vi "Set_Tunnel_Speed.vi"(3 "Mode":T1, 5 "Tunnel Velocity m/s":dbl min=0.0 max=50.0 format="%.2f") -> (0 "Error String":string, 2 "Max allowable Tunnel Velocity":dbl)   [LabVIEW 2017]
doc: "This is an example of using features of the VI Server as a client. It shows how you might browse from one or more applications that may be exporting data from one or more data stations. \n\nThe example shows how to query a server for its list of exported VIs, how to get references to the VIs, and how call them with the Call By Reference function."
uses:
  Sub VIs/ADAM Controls/Tunnel_speed_mode.ctl
  Anemometry/Anemometry Sub Vis/File/Setup_Filetype.ctl
  Sub VIs/ADAM Controls/Update_scan_value.ctl
  Anemometry/Anemometry Sub Vis/Controls/Global_mode.ctl
  Sub VIs/ADAM Controls/Ch_description_ADAM.ctl
  Sub VIs/ADAM Controls/Module_type_ADAM.ctl
  Sub VIs/ADAM Controls/Function_ADAM.ctl
  Sub VIs/ADAM Controls/Channel_State.ctl
  Sub VIs/ADAM Controls/Calib_type_ADAM.ctl
  Sub VIs/ADAM Controls/Address.ctl
  <vilib>/Analysis/baseanly.llb/Mean (DBL).vi
  Anemometry/Anemometry Sub Vis/Globals/Preference_global.vi
  Anemometry/Anemometry Sub Vis/Globals/Trav_pos_global.vi
  Anemometry/Anemometry Sub Vis/Globals/Constants_global.vi
  <vilib>/Analysis/NI_AALBase.lvlib
panel:
  in  "Set EnFlo Tun Speed":refnum<vi>
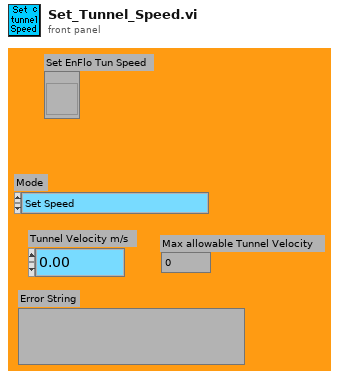
[diagram p1: front panel]
types:
  T1 = typedef "Tunnel_speed_mode.ctl" = enum16{"Set Speed", "Set Speed then wait", "Is tunnel speed allowable?"}
  T2 = typedef "Setup_Filetype.ctl" = enum16{"Measurement Setups", "Calibration Setups", "General", "Results File Plotter Setups", "Speed Calib Tweaks"}
  T3 = typedef "Channel_State.ctl" = enum16{"On", "Off", "Always On", "Always Off"}
  T4 = typedef "Calib_type_ADAM.ctl" = string
  T5 = typedef "Module_type_ADAM.ctl" = string
  T6 = typedef "Ch_description_ADAM.ctl" = cluster{"Ch Name":string, "Type":T5, "Function":T7, "Ch State":T3, "Calibration type":T4, "A":dbl, "B":dbl, "C":dbl, "D":dbl, "Comments":string, "Address":T8, "String":string, "Duty":u16}
  T7 = typedef "Function_ADAM.ctl" = enum16{"Analogue Input", "Digital Input", "Event counter", "Event rate", "Analogue Output", "Digital Output", "Relay Output"}
  T8 = typedef "Address.ctl" = cluster{"Main":i32, "Ch.":i32, "Sub":i32, "Port Name":string}
  T9 = typedef "Global_mode.ctl" = enum16{"Read Global", "Load Global From File", "Write Global to File"}
  T10 = typedef "Update_scan_value.ctl" = cluster{"Channel Name":string, "New Value":dbl}
  T11 = typedef "Server_Comms.ctl" = enum16{"Server Link Healthy", "Do Not Link To Server"}
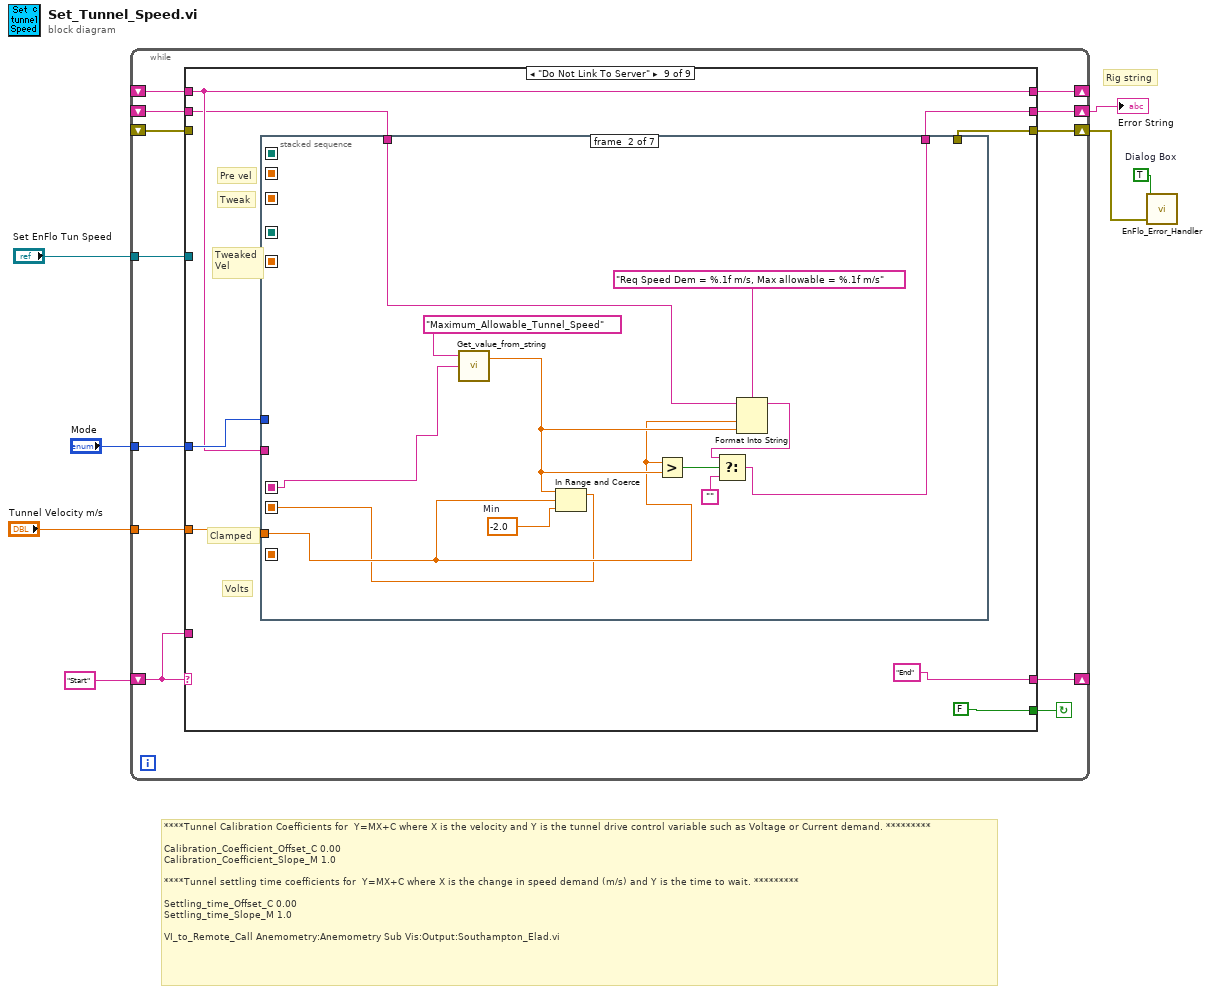
[diagram p0: block diagram]
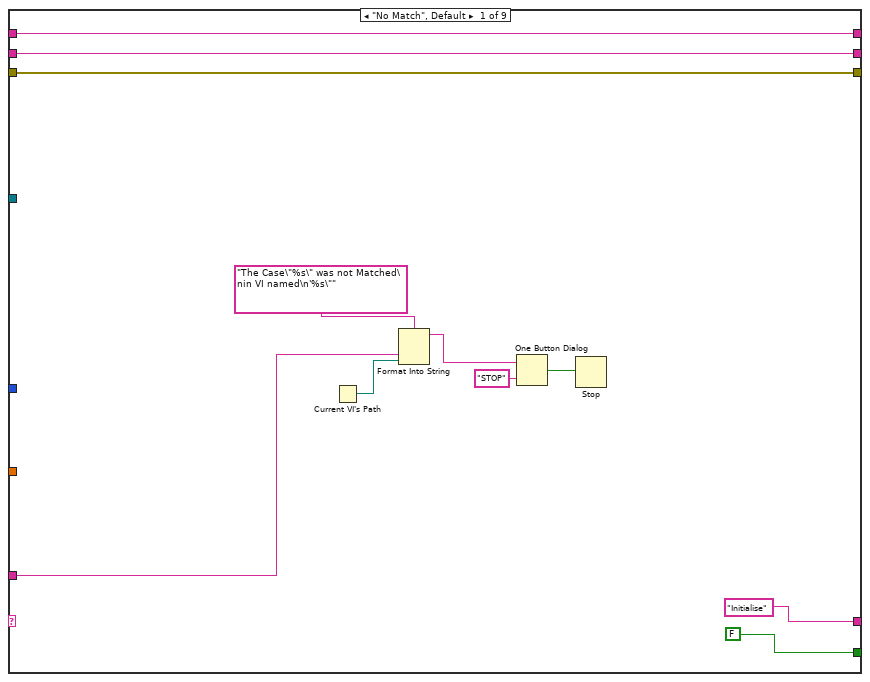
[diagram p2: hidden frame]
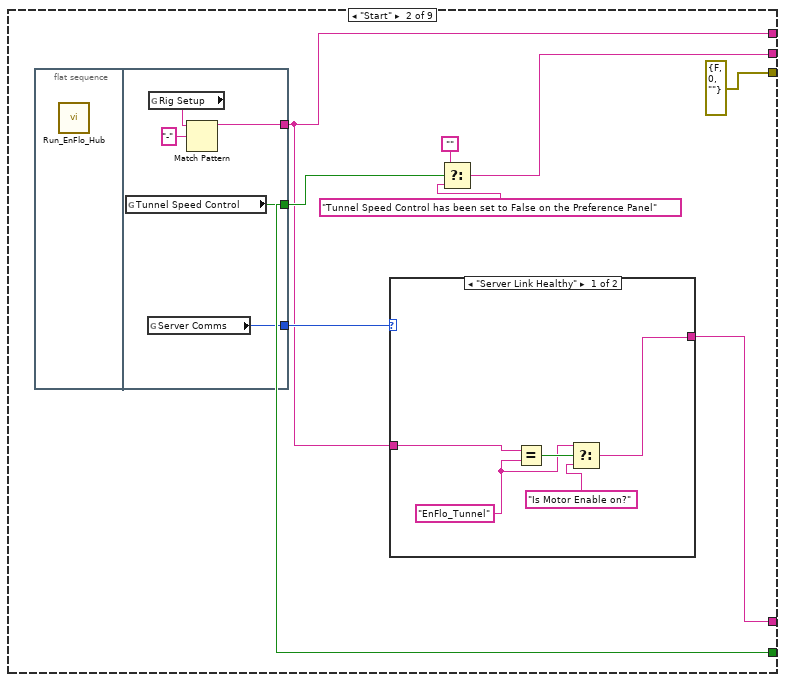
[diagram p3: hidden frame]
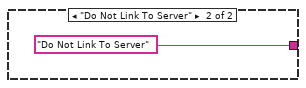
[diagram p4: hidden frame]
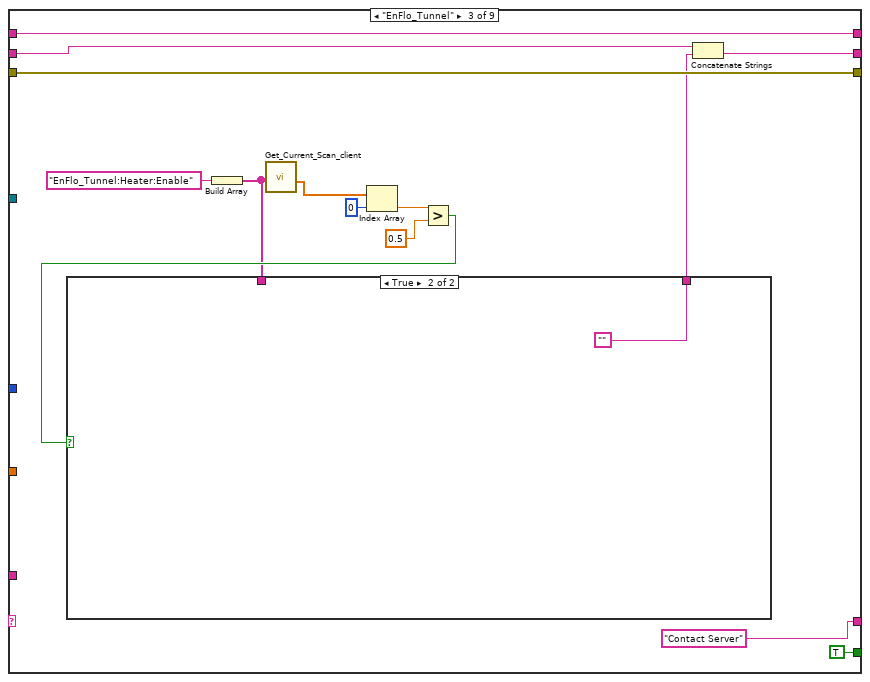
[diagram p5: hidden frame]
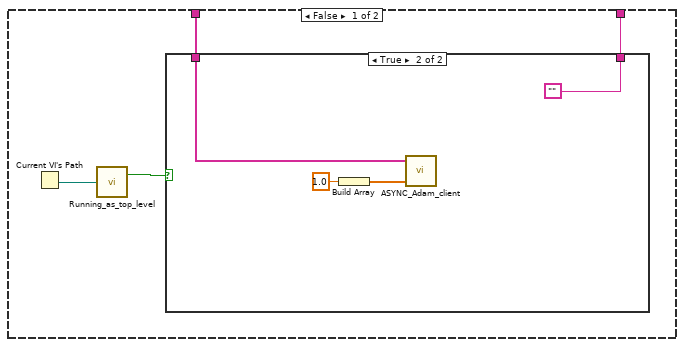
[diagram p6: hidden frame]
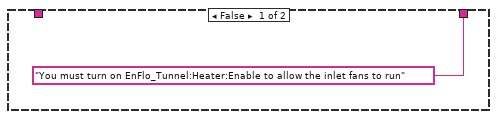
[diagram p7: hidden frame]
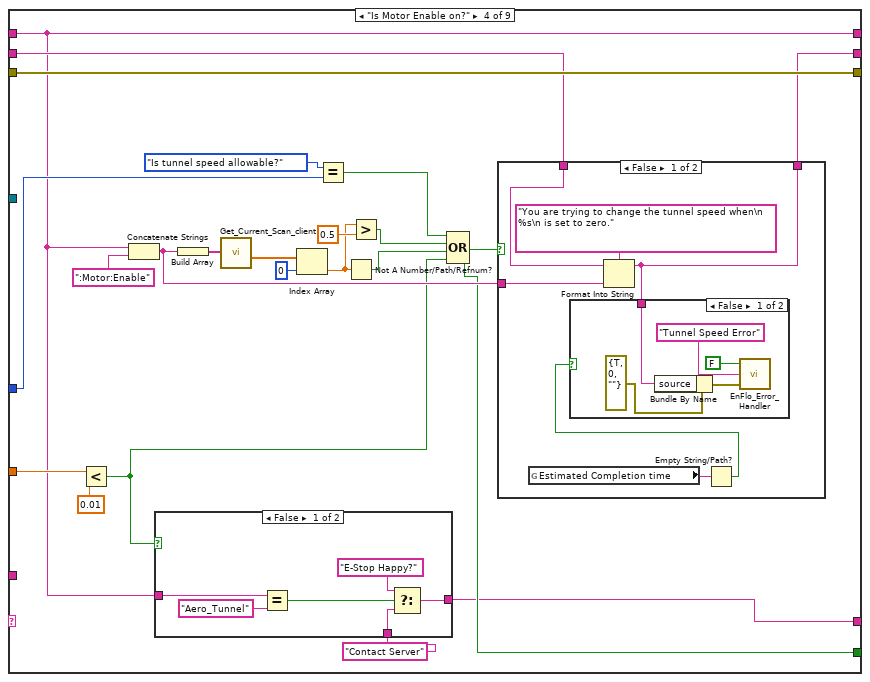
[diagram p8: hidden frame]
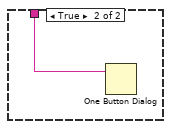
[diagram p10: hidden frame]
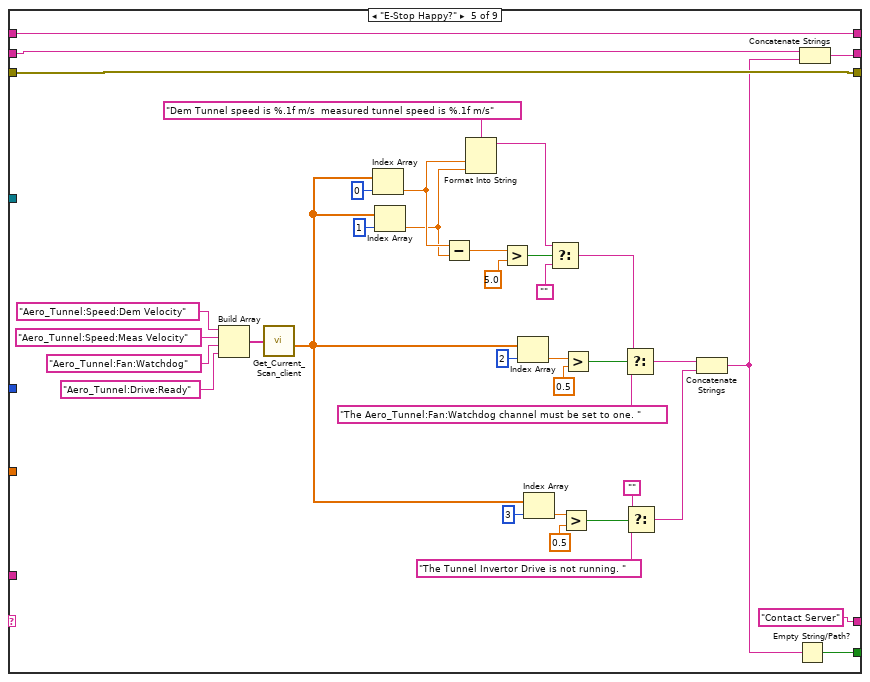
[diagram p12: hidden frame]
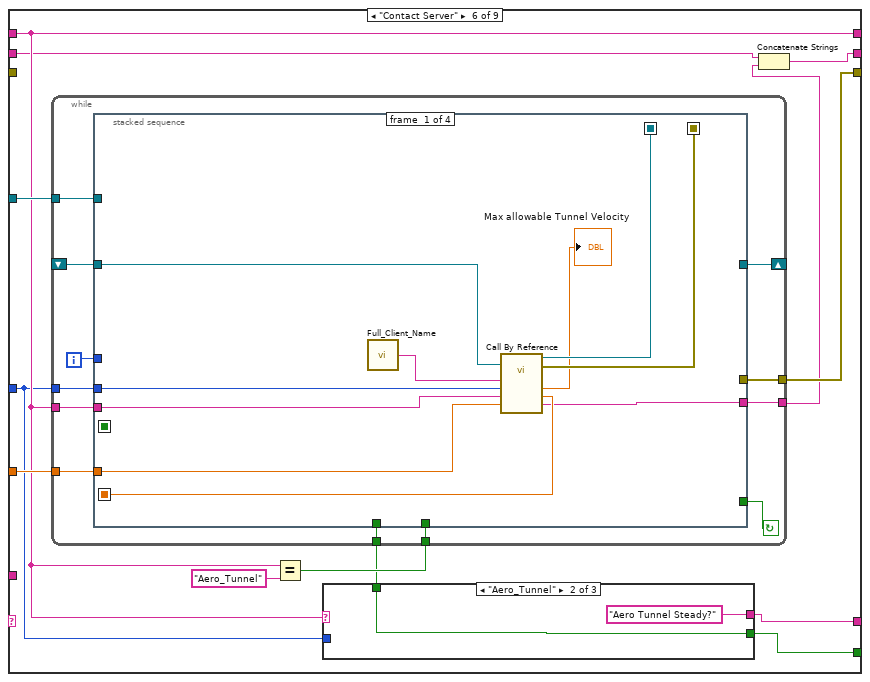
[diagram p13: hidden frame]
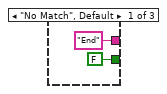
[diagram p14: hidden frame]
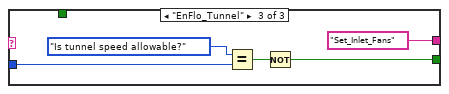
[diagram p15: hidden frame]
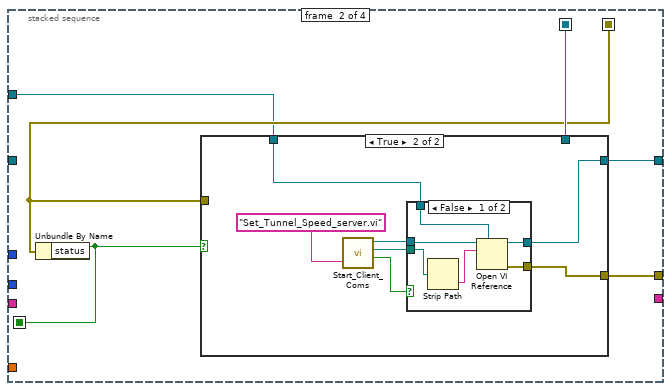
[diagram p16: hidden frame]
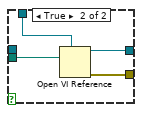
[diagram p18: hidden frame]
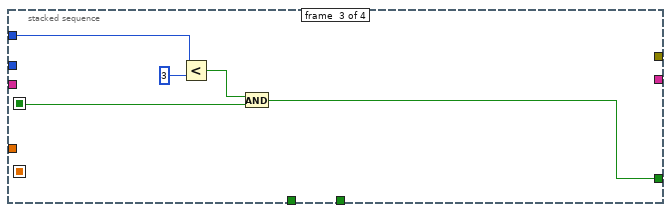
[diagram p19: hidden frame]
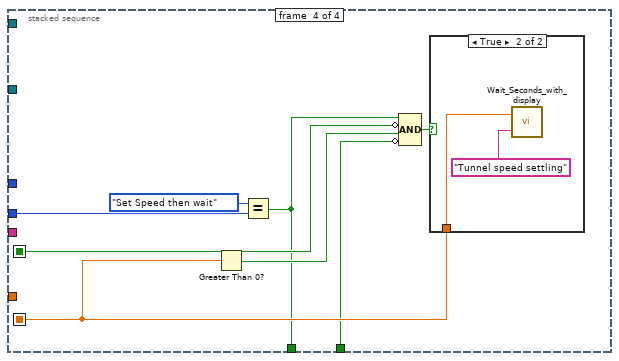
[diagram p20: hidden frame]
diagram:
  w7 = TRUE  # Dialog Box
  # "Rig string"
  # "****Tunnel Calibration Coefficients for  Y=MX+C where X is the velocity and Y is the tunnel drive control variable such as Voltage or Current demand. *********\n\nCalibration_Coefficient_Offset_C\t0.00\nCalibration_Coefficient_Slope_M\t1.0\n\n****Tunnel settling time coefficients for  Y=MX+C where X is the change in speed demand (m/s) and Y is the time to wait. *********\n\nSettling_time_Offset_C\t0.00\nSettling_time_Slope_M\t1.0\n\nVI_to_Remote_Call\tAnemometry:Anemometry Sub Vis:Output:Southampton_Elad.vi"
  n1 = while {
    shift-left: "Start" -> [w18]
    shift-right: [w19] -> _
    shift-right: [w17] -> w5
    shift-left: _ -> [w16]
    shift-right: [w15] -> w4
    shift-left: _ -> [w10]
    tunnel: "Mode" -> [w14]
    tunnel: "Tunnel Velocity m/s" -> [w13]
    shift-right: [w12] -> _
    shift-left: _ -> [w11]
    tunnel: "Set EnFlo Tun Speed" -> [w8]
    stop <- w9 continue-if-true
    n2 = case shown="\"Do Not Link To Server\"" w18 {
      tunnel: [FALSE w36 TRUE ("Tunnel Speed Control") w81 w129 w158 w242 FALSE ("Tunnel Speed Control") FALSE] -> w9
      tunnel: ["Initialise" w32 "Contact Server" ("f") w74 "Contact Server" ("f") w157 "Aero Tunnel Steady?" ("f") "End" ("f") "End"] -> w19
      tunnel: w18 -> [w25 _ _ _ _ _ _ _ _]
      tunnel: [w22 w34 w52 w83 w143 w153 w258 w285 w300] -> w17
      tunnel: w16 -> [w22 _ w54 w82 w144 w154 w258 w285 w297]
      tunnel: [w20 errorcluster {"status"=FALSE, "code"=0, "source"=""} ("error out") w55 w85 w138 w164 w257 w284 w299] -> w15
      tunnel: w14 -> [_ _ _ w79 _ w156 _ _ w302]
      tunnel: w13 -> [_ _ _ w86 _ w165 w249 w266 w301]
      tunnel: [w21 w31 w63 w77 w152 w159 w259 w286 w298] -> w12
      tunnel: w11 -> [w21 _ w63 w77 w152 w159 w259 w286 w298]
      tunnel: w10 -> [w20 _ w55 w85 w138 _ w257 w284 _]
      tunnel: w8 -> [_ _ _ _ _ w163 _ _ _]
      frame "No Match", Default {
        n3 = Current VI's Path() -> (path=w24:path)
        n4 = Format Into String(format string="The Case\"%s\" was not Matched\nin VI named\n'%s\"" ("Format String"), w25, w24) -> (resulting string=w28:string)  [unwired: 2 in, 1 out]
        n5 = One Button Dialog(message=w28, button name ("OK")="STOP") -> (true=w26:bool)
        n6 = Stop(stop? (T)=w26) -> ()
      }
      frame "Start" {
        n7 = flat-sequence {
          tunnel: [w49] -> w38
          tunnel: [w48] -> w36
          tunnel: [w45] -> w31
          frame #0 {
            n8 = call "Run_EnFlo_Hub.vi"() -> ()  [unwired: 1 in, 7 out]
          }
          frame #1 {
            n9 = global read "Preference_global.vi" "Tunnel Speed Control"() -> (w48:bool)
            n10 = global read "Preference_global.vi" "Server Comms"() -> (w49:T11)
            n11 = global read "Preference_global.vi" "Rig Setup"() -> (w47:string)
            n12 = Match Pattern(string=w47, regular expression="-") -> (before substring=w45:string)  [unwired: 4 out]
          }
        }
        n13 = case shown="\"Server Link Healthy\"" w38 {
          tunnel: [w40 "Do Not Link To Server"] -> w32
          tunnel: w31 -> [w43 _]
          frame "Server Link Healthy" {
            w39 = "EnFlo_Tunnel"
            n14 = Equal?(x=w43, y=w39) -> (x = y?=w42:bool)
            n15 = Select(t=w39, s=w42, f="Is Motor Enable on?") -> (s? t:f=w40:string)
          }
          frame "Do Not Link To Server" {
          }
        }
        n16 = Select(t="", s=w36, f="Tunnel Speed Control has been set to False on the Preference Panel" ("Error String")) -> (s? t:f=w34:string)
      }
      frame "EnFlo_Tunnel" {
        n17 = Build Array("EnFlo_Tunnel:Heater:Enable") -> (w56:string[])
        n18 = call "Get_Current_Scan_client.vi"("ADAM Ch Names"=w56) -> ("Numerical Values"=w61:dbl[])  [unwired: 3 out]
        n19 = Index Array(array=w61, index=0) -> (element=w59:dbl)
        n20 = Greater?(x=w59, y=0.5) -> (0:w57:bool)
        n21 = case shown="True" w57 {
          tunnel: w56 -> [w65 _]
          tunnel: [w64 ""] -> w53
          frame False {
            n22 = Current VI's Path() -> (path=w67:path)
            n23 = call "Running_as_top_level.vi"("Vi path name"=w67) -> ("Top Level"=w66:bool)  [unwired: 1 out]
            n24 = case shown="True" w66 {
              tunnel: w65 -> [_ w71]
              tunnel: ["You must turn on EnFlo_Tunnel:Heater:Enable to allow the inlet fans to run" ""] -> w64
              frame False {
              }
              frame True {
                n25 = Build Array(1.0 ("element")) -> (w72:dbl[])
                n26 = call "ASYNC_Adam_client.vi"("Values"=w72, "Channel Names"=w71) -> ()  [unwired: 1 in, 2 out]
              }
            }
          }
          frame True {
          }
        }
        n27 = Concatenate Strings(w54, w53) -> (w52:string)
      }
      frame "Is Motor Enable on?" {
        n28 = Less?(x=w86, y=0.01) -> (x < y?=w76:bool)
        n29 = Concatenate Strings(w77, ":Motor:Enable" ("string")) -> (w84:string)
        n30 = case shown="False" w76 {
          tunnel: w77 -> [w100 _]
          tunnel: [w98 w102] -> w74
          tunnel: "Contact Server" ("f") -> [w96 w102]
          frame False {
            n31 = Equal?(x=w100, y="Aero_Tunnel") -> (x = y?=w99:bool)
            n32 = Select(t="E-Stop Happy?" ("f"), s=w99, f=w96) -> (s? t:f=w98:string)
          }
          frame True {
          }
        }
        n33 = Build Array(w84) -> (w88:string[])
        n34 = call "Get_Current_Scan_client.vi"("ADAM Ch Names"=w88) -> ("Numerical Values"=w89:dbl[])  [unwired: 3 out]
        n35 = Index Array(array=w89, index=0) -> (element=w91:dbl)
        n36 = Equal?(x=Tunnel_speed_mode."Is tunnel speed allowable?" ("Mode"), y=w79) -> (x = y?=w78:bool)
        n37 = Not A Number/Path/Refnum?(number/path/refnum=w91) -> (NaN/Path/Refnum?=w93:bool)
        n38 = Greater?(x=w91, y=0.5) -> (0:w94:bool)
        n39 = Compound Arithmetic op=OR(w78, w94, w93, w76) -> (w81:bool)
        n40 = case shown="False" w81 {
          tunnel: w84 -> [w107 _]
          tunnel: [w104 w115] -> w83
          tunnel: w82 -> [w103 w115]
          frame False {
            n41 = global read "Trav_pos_global.vi" "Estimated Completion time"() -> (w106:string)
            n42 = Format Into String(format string="You are trying to change the tunnel speed when\n %s\n is set to zero.", initial string=w103, w107) -> (resulting string=w104:string)  [unwired: 1 in, 1 out]
            n43 = Empty String/Path?(string/path=w106) -> (empty?=w105:bool)
            n44 = case shown="False" w105 {
              tunnel: w104 -> [w110 w114]
              frame False {
                n45 = Bundle By Name(cluster=errorcluster {"status"=TRUE, "code"=0, "source"=""} ("error in (no error)"), "source"=w110) -> (w111:errorcluster)
                n46 = call "EnFlo_Error_Handler.vi"("error in (no error)"=w111, "Error Type"="Tunnel Speed Error", "Dialog Box (T)"=FALSE) -> ()  [unwired: 3 out]
              }
              frame True {
                n47 = One Button Dialog(message=w114) -> ()  [unwired: 2 out]
              }
            }
          }
          frame True {
          }
        }
      }
      frame "E-Stop Happy?" {
        n48 = Build Array("Aero_Tunnel:Speed:Dem Velocity", "Aero_Tunnel:Speed:Meas Velocity", "Aero_Tunnel:Fan:Watchdog", "Aero_Tunnel:Drive:Ready") -> (w149:string[])
        n49 = call "Get_Current_Scan_client.vi"("ADAM Ch Names"=w149) -> ("Numerical Values"=w126:dbl[])  [unwired: 1 in, 2 out]
        n50 = Index Array(array=w126, index=0) -> (element=w142:dbl)
        n51 = Index Array(array=w126, index=1) -> (element=w141:dbl)
        n52 = Subtract(x=w142, y=w141) -> (x-y=w146:dbl)
        n53 = Format Into String(format string="Dem Tunnel speed is %.1f m/s  measured tunnel speed is %.1f m/s", w142, w141) -> (resulting string=w139:string)  [unwired: 2 in, 1 out]
        n54 = Greater?(x=w146, y=5.0) -> (0:w136:bool)
        n55 = Index Array(array=w126, index=2) -> (element=w133:dbl)
        n56 = Index Array(array=w126, index=3) -> (element=w125:dbl)
        n57 = Select(t=w139, s=w136, f="") -> (s? t:f=w131:string)
        n58 = Greater?(x=w125, y=0.5) -> (0:w123:bool)
        n59 = Greater?(x=w133, y=0.5) -> (0:w116:bool)
        n60 = Select(t=w131, s=w116, f="The Aero_Tunnel:Fan:Watchdog channel must be set to one. ") -> (s? t:f=w120:string)
        n61 = Select(t="", s=w123, f="The Tunnel Invertor Drive is not running. ") -> (s? t:f=w119:string)
        n62 = Concatenate Strings(w120, w119) -> (w118:string)
        n63 = Empty String/Path?(string/path=w118) -> (empty?=w129:bool)
        n64 = Concatenate Strings(w144, w118) -> (w143:string)
      }
      frame "Contact Server" {
        n65 = Equal?(x=w159, y="Aero_Tunnel") -> (x = y?=w161:bool)
        n66 = while {
          tunnel: w156 -> [w181]
          tunnel: w165 -> [w182]
          tunnel: [w183] -> w164
          shift-left: _ -> [w178]
          shift-right: [w186] -> _
          tunnel: [w180] -> w155
          tunnel: w159 -> [w179]
          tunnel: w163 -> [w177]
          tunnel: w161 -> [w176]
          tunnel: [w175] -> w160
          i -> [w185]
          stop <- w184 continue-if-true
          n67 = stacked-sequence {
            seq-local: [w195 _ _ _] -> [_ w201 _ _]
            seq-local: [w194 _ _ _] -> [_ w199 _ _]
            seq-local: [_ w200 _ _] -> [_ _ w223 w230]
            seq-local: [w191 _ _ _] -> [_ _ _ w233]
            tunnel: w178 -> [w196 _ _ _]
            tunnel: [_ w202 _ _] -> w186
            tunnel: w185 -> [_ _ w224 _]
            tunnel: [_ _ w222 _] -> w184
            tunnel: [_ w198 _ _] -> w183
            tunnel: w182 -> [w192 _ _ _]
            tunnel: w181 -> [w188 _ _ w234]
            tunnel: [w190 _ _ _] -> w180
            tunnel: w179 -> [w189 _ _ _]
            tunnel: w177 -> [_ w197 _ _]
            tunnel: w176 -> [_ _ _ w228]
            tunnel: [_ _ _ w227] -> w175
            frame #0 {
              n68 = call "Full_Client_Name.vi"() -> ("Client Name"=w193:string)
              n69 = call-by-ref "?"(reference=w196, "Tunnel Velocity m/s"=w192, "Rig Name"=w189, "Mode"=w188, "Client Name"=w193) -> (reference out=w195:refnum<vi>, error out=w194:errorcluster, "Error String"=w190:string, "Settling Time (s)"=w191:dbl, "Max allowable Tunnel Velocity"=→"Max allowable Tunnel Velocity":dbl)  [unwired: 1 in, 1 out]
            }
            frame #1 {
              n70 = Unbundle By Name(w199) -> ("status"=w200:bool)
              n71 = case shown="True" w200 {
                tunnel: [w203 w207] -> w202
                tunnel: w201 -> [w203 _]
                tunnel: [w204 w206] -> w198
                tunnel: w199 -> [w204 _]
                tunnel: w197 -> [_ w205]
                frame False {
                }
                frame True {
                  n72 = call "Start_Client_Coms.vi"("VI name to run on server"="Set_Tunnel_Speed_server.vi") -> ("LabVIEW application reference"=w209:refnum<vi>, "Checked VI name"=w210:path, "Local Call"=w208:bool)  [unwired: 1 in, 1 out]
                  n73 = case shown="False" w208 {
                    tunnel: [w216 w221] -> w207
                    tunnel: w205 -> [w214 w220]
                    tunnel: w210 -> [w213 w219]
                    tunnel: w209 -> [w212 _]
                    tunnel: [w215 w218] -> w206
                    frame False {
                      n74 = Strip Path(path=w213) -> (name=w217:string)  [unwired: 1 out]
                      n75 = Open VI Reference(type specifier VI Refnum (for type only)=w214, application reference (local)=w212, vi path=w217) -> (vi reference=w216:refnum<vi>, error out=w215:errorcluster)  [unwired: 1 in, 2 out]
                    }
                    frame True {
                      n76 = Open VI Reference(type specifier VI Refnum (for type only)=w220, vi path=w219) -> (vi reference=w221:refnum<vi>, error out=w218:errorcluster)  [unwired: 1 in, 3 out]
                    }
                  }
                }
              }
            }
            frame #2 {
              n77 = Less?(x=w224, y=3) -> (x < y?=w226:bool)
              n78 = And(x=w226, y=w223) -> (x .and. y?=w222:bool)
            }
            frame #3 {
              n79 = Greater Than 0?(x=w233) -> (x > 0?=w229:bool)
              n80 = Equal?(x=Tunnel_speed_mode."Set Speed then wait" ("Mode"), y=w234) -> (x = y?=w227:bool)
              n81 = Compound Arithmetic op=AND(w227, invert w230, w229, invert w228) -> (w231:bool)
              n82 = case shown="True" w231 {
                tunnel: w233 -> [_ w235]
                frame False {
                }
                frame True {
                  n83 = call "Wait_Seconds_with_display.vi"("Message"="Tunnel speed settling", "Seconds to wait"=w235) -> ()  [unwired: 2 out]
                }
              }
            }
          }
        }
        n84 = case shown="\"Aero_Tunnel\"" w159 {
          tunnel: w160 -> [_ w168 _]
          tunnel: [FALSE w168 w170] -> w158
          tunnel: ["End" ("f") "Aero Tunnel Steady?" ("f") "Set_Inlet_Fans" ("f")] -> w157
          tunnel: w156 -> [_ _ w172]
          frame "No Match", Default {
          }
          frame "Aero_Tunnel" {
          }
          frame "EnFlo_Tunnel" {
            n85 = Equal?(x=Tunnel_speed_mode."Is tunnel speed allowable?" ("Mode"), y=w172) -> (x = y?=w171:bool)
            n86 = Not(x=w171) -> (.not. x?=w170:bool)
          }
        }
        n87 = Concatenate Strings(w154, w155) -> (w153:string)
      }
      frame "Aero Tunnel Steady?" {
        n88 = call "Get_Ch_Time_Trace.vi"("Desired Ch Names"=string[] ["Aero_Tunnel:Fan:RPM", "Aero_Tunnel:Speed:Dem Velocity"] ("ADAM Ch Names"), "History Length (mins)"=0.3) -> ("Output array"=w252:dbl[][])  [unwired: 2 out]
        n89 = Index Array(array=w252, index (row)=0) -> (element=w248:dbl[])  [unwired: 1 in]
        n90 = Index Array(array=w252, index (row)=1) -> (element=w251:dbl[])  [unwired: 1 in]
        n91 = call-poly <vilib>:"Mean.vi"("X"=w251) -> ("mean"=w250:dbl)  [unwired: 1 out]
        n92 = Array Max & Min(array=w248) -> (max value=w247:dbl, min value=w246:dbl)  [unwired: 2 out]
        n93 = Subtract(x=w250, y=w249) -> (x-y=w239:dbl)
        n94 = Subtract(x=w247, y=w246) -> (x-y=w245:dbl)
        n95 = In Range and Coerce(upper limit=0.01, x=w239, lower limit=-0.01) -> (In Range?=w238:bool)  [unwired: 1 out]
        n96 = Greater?(x=w245, y=7.0) -> (0:w243:bool)
        n97 = Not(x=w238) -> (.not. x?=w237:bool)
        n98 = Or(x=w243, y=w237) -> (x .or. y?=w242:bool)
        n99 = case shown="True" w242 {
          frame False {
          }
          frame True {
            n100 = call "Wait_Seconds_with_display.vi"("Message"="Tunnel speed settling", "Seconds to wait"=4.0) -> ()  [unwired: 2 out]
          }
        }
      }
      frame "Set_Inlet_Fans" {
        w263 = FALSE  # Delete First Rows?
        n101 = global read "Constants_global.vi" "All_Users"() -> (w271:path)
        n102 = Build Path(base path=w271, name or relative path="Inlet_Fan_Settings.xls") -> (appended path=w273:path)
        n103 = call "Read_Data_file.vi"("Results file"=w273, "Delete First Rows?"=w263) -> ("Ch names Out"=w279:string[], "Channel Values Out"=w275:string[][], "mark after read (chars.)"=w265:i32)  [unwired: 7 in, 8 out]
        n104 = Array Subset(array=w279, index=1) -> (w267:string[])  [unwired: 1 in]
        n105 = Array Subset(array=w275, index (col)=1 ("index")) -> (w270:string[][])  [unwired: 3 in]
        n106 = Index Array(array=w275, index (col)=0 ("index (row)")) -> (element=w277:string[])  [unwired: 1 in]
        n107 = Fract/Exp String To Number(string=w277) -> (number=w278:dbl[])  [unwired: 3 in, 1 out]
        n108 = Transpose 2D Array(2D array=w270) -> (transposed array=w269:string[][])
        n109 = Threshold 1D Array(2:w266, 3:w278) -> (0:w281:dbl)  [unwired: 1 in]
        n110 = for {
          tunnel: w269 -> [w296] mode=indexing
          tunnel: w281 -> [w295]
          tunnel: [w289] -> w268 mode=indexing
          n111 = Fract/Exp String To Number(string=w296) -> (number=w294:dbl[])  [unwired: 3 in, 1 out]
          n112 = Interpolate 1D Array(1:w295, 2:w294) -> (0:w291:dbl)
          n113 = Greater?(x=w291, y=2.5) -> (0:w292:bool)
          n114 = Select(t=w291, s=w292, f=0.0) -> (s? t:f=w289:dbl)
        }
        n115 = Greater Than 0?(x=w265) -> (x > 0?=w264:bool)
        n116 = case shown="True" w264 {
          tunnel: w268 -> [_ w288]
          tunnel: w267 -> [_ w287]
          frame False {
          }
          frame True {
            n117 = call "ASYNC_Adam_client.vi"("Values"=w288, "Channel Names"=w287) -> ()  [unwired: 1 in, 2 out]
          }
        }
      }
      frame "Do Not Link To Server" {
        # "Clamped"
        # "Pre vel"
        # "Tweak"
        # "Tweaked\nVel"
        # "Volts"
        n118 = stacked-sequence {
          seq-local: [w311 _ _ _ _ _ _] -> [_ w326 w332 w340 w355 w414 _]
          seq-local: [_ _ w327 _ _ _ _] -> [_ _ _ _ w359 _ _]
          seq-local: [_ _ _ w336 _ _ _] -> [_ _ _ _ w354 _ w427]
          seq-local: [_ _ _ w339 _ _ _] -> [_ _ _ _ w357 w409 _]
          seq-local: [_ _ _ _ w356 _ _] -> [_ _ _ _ _ w408 _]
          seq-local: [_ _ _ w341 _ _ _] -> [_ _ _ _ _ _ w433]
          seq-local: [w308 _ _ _ _ _ _] -> [_ _ _ _ _ _ w435]
          seq-local: [_ w317 _ _ _ _ _] -> [_ _ _ w334 _ _ w432]
          tunnel: w301 -> [_ w318 _ _ _ _ _]
          tunnel: w298 -> [w312 _ _ w348 _ _ w429]
          tunnel: w302 -> [_ _ _ _ w358 w403 _]
          tunnel: [_ w316 _ _ _ _ _] -> w300
          tunnel: [_ _ _ _ w353 _ _] -> w299
          tunnel: w297 -> [_ w315 _ _ _ _ _]
          frame #0 {
            n119 = Concatenate Strings(w312, "_Calib" ("Substring"), ".xls" ("string")) -> (w306:string)
            n120 = call "Setup_Filepath.vi"("Setup File Type"=Setup_Filetype."Speed Calib Tweaks", "Filename in"=w306) -> ("Filename Out"=w305:path)  [unwired: 1 out]
            n121 = call "Setup_Filepath.vi"("Setup File Type"=Setup_Filetype."Speed Calib Tweaks", "Filename in"="Current_Values.xls" ("name or relative path")) -> ("Filename Out"=w308:path)  [unwired: 1 out]
            n122 = call "Read_File_No_Error.vi"("Filename"=w305) -> ("string"=w311:string)  [unwired: 2 in, 7 out]
          }
          frame #1 {
            w320 = -2.0  # Min
            n123 = call "Get_value_from_string.vi"("Input string"=w326, "Variable name"="Maximum_Allowable_Tunnel_Speed") -> ("Value"=w319:dbl)  [unwired: 1 in, 1 out]
            n124 = In Range and Coerce(upper limit=w319, x=w318, lower limit=w320) -> (coerced(x)=w317:dbl)  [unwired: 1 out]
            n125 = Greater?(x=w318, y=w319) -> (0:w321:bool)
            n126 = Format Into String(format string="Req Speed Dem = %.1f m/s, Max allowable = %.1f m/s", initial string=w315, w318, w319) -> (resulting string=w323:string)  [unwired: 1 in, 1 out]
            n127 = Select(t=w323, s=w321, f="") -> (s? t:f=w316:string)
          }
          frame #2 {
            n128 = call "Get_Characters_from_string.vi"("Input string"=w332, "Variable name"="VI_to_Remote_Call") -> ("Value"=w330:string)  [unwired: 1 in, 1 out]
            n129 = global read "Constants_global.vi" "EnFlo SW Folder"() -> (w328:path)
            n130 = call "String_to_Pathname.vi"("Input String"=w330) -> ("path"=w331:path)
            n131 = Path to Array of Strings(0:w331) -> (2:w329:string[])  [unwired: 1 out]
            n132 = call "Build_Pathname.vi"("PathElements"=w329, "PathnameIn"=w328) -> ("AppendedPath"=w327:path)
          }
          frame #3 {
            n133 = local write "Tunnel Velocity m/s"(w334) -> ()
            n134 = call "Add_to_speed_calib_file.vi"("Desired Velocity"=w334, "Rig Name"=w348, "Mode"=enum16{"Add Row", "Get Error Value"}."Get Error Value") -> ("Tweaked Demand"=w339:dbl, "Calib Tweak %"=w341:dbl)  [unwired: 3 in]
            n135 = Less?(x=w339, y=0.01) -> (x < y?=w337:bool)
            n136 = call "Get_value_from_string.vi"("Input string"=w340, "Variable name"="Calibration_Coefficient_Offset_C") -> ("Value"=w342:dbl)  [unwired: 1 in, 1 out]
            n137 = call "Get_value_from_string.vi"("Input string"=w340, "Variable name"="Calibration_Coefficient_Slope_M") -> ("Value"=w344:dbl)  [unwired: 1 in, 1 out]
            n138 = Multiply(x=w344, y=w339) -> (x*y=w343:dbl)
            n139 = Add(x=w342, y=w343) -> (x+y=w335:dbl)
            n140 = case shown="False" w337 {
              tunnel: w340 -> [_ w351]
              tunnel: [w349 w350] -> w336
              tunnel: w335 -> [w349 _]
              frame False {
              }
              frame True {
                n141 = call "Get_value_from_string.vi"("Input string"=w351, "Variable name"="Zero_Velocity_Output_Voltage") -> ("Value"=w350:dbl)  [unwired: 1 in, 1 out]
              }
            }
          }
          frame #4 {
            n142 = while {
              tunnel: w359 -> [w369]
              tunnel: w358 -> [w368]
              tunnel: w357 -> [w367]
              tunnel: [w366] -> w356
              shift-right: [w364] -> _
              shift-left: _ -> [w363]
              tunnel: [w362] -> w353
              tunnel: w355 -> [w361]
              tunnel: w354 -> [w360]
              stop <- TRUE stop-if-true
              n143 = case shown="\"Set Speed then wait\", Default" w368 {
                tunnel: w369 -> [_ w389]
                tunnel: w367 -> [_ w376]
                tunnel: [w371 w378] -> w366
                tunnel: [w371 w376] -> w364
                tunnel: w363 -> [w371 w377]
                tunnel: [errorcluster {"status"=FALSE, "code"=0, "source"=""} ("error out") w372] -> w362
                tunnel: w361 -> [_ _]
                tunnel: w360 -> [_ w375]
                frame "Is tunnel speed allowable?" {
                }
                frame "Set Speed then wait", Default {
                  n144 = Open VI Reference(type specifier VI Refnum (for type only)=refnum<vi> refnum, vi path=w389) -> (vi reference=w387:refnum<vi>, error out=w386:errorcluster)  [unwired: 1 in, 3 out]
                  n145 = property class="VI Interface Type 0"(reference=w387, error in=w386) -> (reference out=w384:refnum<vi>, error out=w385:errorcluster, "Front Panel.Open"=w383:bool)
                  n146 = case shown="False" w383 {
                    tunnel: w385 -> [w394 w397]
                    tunnel: w384 -> [w393 w398]
                    tunnel: [w392 w398] -> w382
                    tunnel: [w391 w397] -> w381
                    tunnel: [0.0 ("Tweaked Demand") w396] -> w378
                    tunnel: w377 -> [_ w396]
                    frame False {
                      n147 = property class="VI Interface Type 0"(reference=w393, error in=w394, "Front Panel.Open"=TRUE ("Front Panel Window:Open")) -> (reference out=w392:refnum<vi>, error out=w391:errorcluster)
                    }
                    frame True {
                    }
                  }
                  n148 = call-by-ref "?"(reference=w382, error in=w381, "Demand"=w375) -> (reference out=w379:refnum<vi>, error out=w380:errorcluster, "error out"=w373:errorcluster)
                  n149 = Close Reference(reference=w379, error in (no error)=w380) -> (error out=w374:errorcluster)
                  n150 = Select(t=w374, s=w374, f=w373) -> (s? t:f=w372:errorcluster)
                }
              }
            }
          }
          frame #5 {
            n151 = Subtract(x=w408, y=w409) -> (x-y=w407:dbl)
            n152 = Absolute Value(x=w407) -> (abs(x)=w401:dbl)
            n153 = call "Get_value_from_string.vi"("Input string"=w414, "Variable name"="Settling_time_Offset_C") -> ("Value"=w410:dbl)  [unwired: 1 in, 1 out]
            n154 = call "Get_value_from_string.vi"("Input string"=w414, "Variable name"="Settling_time_Slope_M") -> ("Value"=w412:dbl)  [unwired: 1 in, 1 out]
            n155 = Multiply(x=w412, y=w401) -> (x*y=w411:dbl)
            n156 = Add(x=w410, y=w411) -> (x+y=w402:dbl)
            n157 = Greater?(x=w401, y=0.05) -> (0:w399:bool)
            n158 = Equal?(x=Tunnel_speed_mode."Set Speed then wait" ("Mode"), y=w403) -> (x = y?=w405:bool)
            n159 = Compound Arithmetic op=AND(w399, w405) -> (w404:bool)
            n160 = case shown="False" w404 {
              tunnel: w402 -> [_ w416]
              frame False {
              }
              frame True {
                n161 = call "Wait_Seconds_with_display.vi"("Message"="Tunnel speed settling", "Seconds to wait"=w416) -> ()  [unwired: 2 out]
              }
            }
          }
          frame #6 {
            n162 = Concatenate Strings(w429, ":Speed:Dem_Voltage" ("string")) -> (w424:string)
            n163 = Bundle By Name(cluster=T6 {"Ch Name"="", "Type"="", "Function"=enum."Analogue Input", "Ch State"=enum."On", "Calibration type"="", "A"=0.0, "B"=0.0, "C"=0.0, "D"=0.0, "Comments"="", "Address"={"Main"=0, "Ch."=0, "Sub"=0, "Port Name"=""}, "String"="", "Duty"=0} ("Ch Discription"), "Ch Name"=w424, "Type"=T5 "Hold Value", "Calibration type"=T4 "", "Ch State"=Channel_State."On") -> (w418:T6)
            n164 = Bundle By Name(cluster=T10 {"Channel Name"="", "New Value"=0.0} ("Update Scan Value Cluster"), "Channel Name"=w424, "New Value"=w427) -> (w430:T10)
            n165 = call "Value_to_string.vi"("Value"=w433, "Label for value"="Calib Tweak") -> ("Output string"=w438:string)  [unwired: 1 in]
            n166 = call "Value_to_string.vi"("Value"=w432, "Label for value"="Velocity Demand") -> ("Output string"=w437:string)  [unwired: 1 in]
            n167 = Concatenate Strings(w438, w437) -> (w436:string)
            n168 = call "Write_File_Simple.vi"("append to file? (new file:F)"=FALSE, "character string"=w436, "file path"=w435) -> ()  [unwired: 2 out]
            n169 = Build Array(w418) -> (w419:T6[])
            n170 = Build Array(w430) -> (w420:T10[])
            n171 = call "Read_Write_Local_table.vi"("Mode"=Global_mode."Write Global to File", "Ch Values in"=w420, "Channels Descriptions In"=w419) -> ()  [unwired: 3 out]
          }
        }
      }
    }
  }
  "Error String" <- w5
  n172 = call "EnFlo_Error_Handler.vi"("error in (no error)"=w4, "Dialog Box (T)"=w7) -> ()  [unwired: 1 in, 3 out]
